vi "Revision Query.vi"(8 "error in (no error)":errorcluster, 11 "VISA resource name":refnum<visa-resource-name>) -> (0 "error out":errorcluster, 1 "Instr Serial Number":string, 2 "Instr Firmware Revision":string, 3 "VISA resource name out":refnum<visa-resource-name>, 4 "Instr Model Number":string, 5 "Instrument Driver Revision":string, 6 "Option Card Serial Number":string)   [LabVIEW 2012, in "Lake Shore 336.lvlib"]
doc: "Queries the current instrument firmware revision and instrument driver revision.\n\nFor detailed driver information including modification history, refer to the Readme file."
uses:
  Lake Shore 336.lvlib
  Instance           1 22Saved   Revision Query .vi
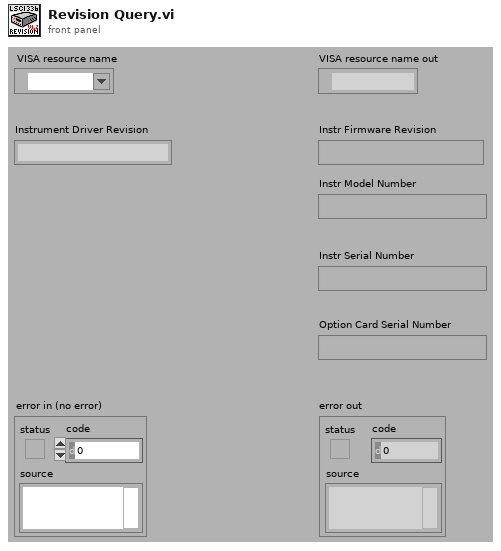
[diagram p1: front panel]
types:
  T1 = enum32{"invalid app kind", "Development System", "Run Time System", "Student Edition", "Embedded LabVIEW", "Evaluation", "Custom"}
  T2 = cluster{"Major":u16, "Minor":u16, "Fix":u16, "Build":u16}
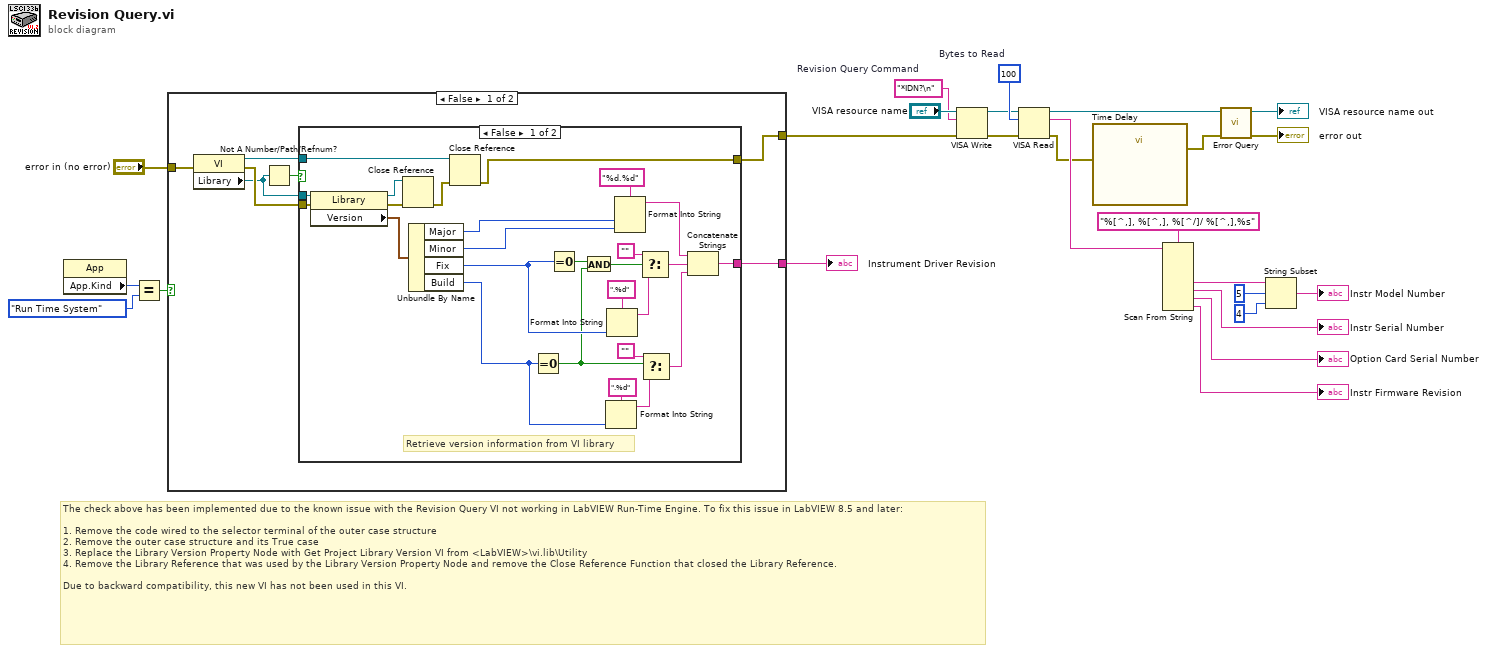
[diagram p0: block diagram]
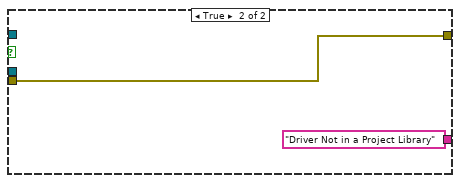
[diagram p2: hidden frame]
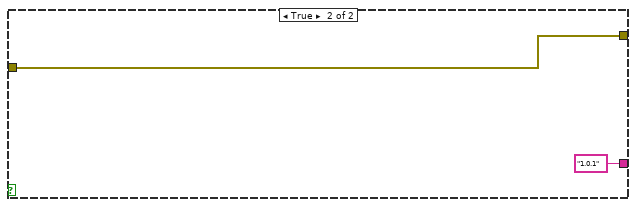
[diagram p3: hidden frame]
diagram:
  w21 = "*IDN?\n"  # Revision Query Command
  w24 = u32 100  # Bytes to Read
  # "The check above has been implemented due to the known issue with the Revision Query VI not working in LabVIEW Run-Time Engine. To fix this issue in LabVIEW 8.5 and later:\n\n1. Remove the code wired to the selector terminal of the outer case structure\n2. Remove the outer case structure and its True case\n3. Replace the Library Version Property Node with Get Project Library Version VI from <LabVIEW>\\vi.lib\\Utility\n4. Remove the Library Reference that was used by the Library Version Property Node and remove the Close Reference Function that closed the Library Reference.\n\nDue to backward compatibility, this new VI has not been used in this VI."
  n1 = property class="App"() -> ("App.Kind"=w4:T1)  [unwired: 2 in, 2 out]
  n2 = Equal?(x=w4, y=T1."Run Time System") -> (x = y?=w2:bool)
  n3 = case shown="False" w2 {
    tunnel: [w28 "1.0.1"] -> w17
    tunnel: "error in (no error)" -> [w27 w61]
    tunnel: [w26 w61] -> w16
    frame False {
      n4 = property on="Property Node" class="VI"(error in=w27) -> (reference out=w32:refnum<vi>, error out=w31:errorcluster, "Library"=w30:refnum<vi>)  [unwired: 1 in]
      n5 = Not A Number/Path/Refnum?(number/path/refnum=w30) -> (NaN/Path/Refnum?=w29:bool)
      n6 = case shown="False" w29 {
        tunnel: w32 -> [w55 _]
        tunnel: w31 -> [w40 w60]
        tunnel: [w35 w60] -> w26
        tunnel: [w34 "Driver Not in a Project Library"] -> w28
        tunnel: w30 -> [w33 _]
        frame False {
          # "Retrieve version information from VI library"
          n7 = property on="Property Node" class="Library"(reference=w33, error in=w40) -> (reference out=w57:refnum<vi>, error out=w58:errorcluster, "Version"=w54:T2)
          n8 = Close Reference(reference=w57, error in (no error)=w58) -> (error out=w56:errorcluster)
          n9 = Unbundle By Name(w54) -> ("Major"=w43:u16, "Minor"=w42:u16, "Fix"=w39:u16, "Build"=w41:u16)
          n10 = Close Reference(reference=w55, error in (no error)=w56) -> (error out=w35:errorcluster)
          n11 = Equal To 0?(x=w41) -> (x = 0?=w37:bool)
          n12 = Equal To 0?(x=w39) -> (x = 0?=w38:bool)
          n13 = And(x=w38, y=w37) -> (x .and. y?=w36:bool)
          n14 = Format Into String(format string=".%d", w41) -> (resulting string=w47:string)  [unwired: 2 in, 1 out]
          n15 = Format Into String(format string=".%d", w39) -> (resulting string=w51:string)  [unwired: 2 in, 1 out]
          n16 = Format Into String(format string="%d.%d", w43, w42) -> (resulting string=w49:string)  [unwired: 2 in, 1 out]
          n17 = Select(t="" ("Empty String Constant"), s=w36, f=w51) -> (s? t:f=w48:string)
          n18 = Select(t="" ("Empty String Constant"), s=w37, f=w47) -> (s? t:f=w44:string)
          n19 = Concatenate Strings(w49, w48, w44) -> (w34:string)
        }
        frame True {
        }
      }
    }
    frame True {
    }
  }
  "Instrument Driver Revision" <- w17
  n20 = VISA Write(VISA resource name="VISA resource name", write buffer=w21, error in (no error)=w16) -> (VISA resource name out=w23:refnum<visa-resource-name>, error out=w22:errorcluster)  [unwired: 1 out]
  n21 = VISA Read(VISA resource name=w23, byte count=w24, error in (no error)=w22) -> (VISA resource name out=w20:refnum<visa-resource-name>, read buffer=w12:string, error out=w10:errorcluster)  [unwired: 1 out]
  n22 = call "Time Delay"("error in (no error)"=w10) -> ("error out"=w9:errorcluster)  [unwired: 10 in]
  n23 = Scan From String(format string="%[^,], %[^,], %[^/]/ %[^,],%s", input string=w12) -> (output 2=w5:string, output 3=→"Instr Serial Number":string, output 4=→"Option Card Serial Number":string, output 5=→"Instr Firmware Revision":string)  [unwired: 8 in, 3 out]
  n24 = call "Error Query.vi"("error in (no error)"=w9, "VISA resource name"=w20) -> ("error out"=→"error out":errorcluster, "VISA resource name out"=→"VISA resource name out":refnum<visa-resource-name>)  [unwired: 7 in, 1 out]
  n25 = String Subset(string=w5, offset (0)=5, length (rest)=4) -> (substring=→"Instr Model Number":string)
